vi "Get Section.vi"(11 "Device Info in":refnum<class "Device Info.lvclass">) -> (2 "Section":string, 3 "Device Info out":refnum<class "Device Info.lvclass">)   [LabVIEW 2024, in "EDS.lvlib" / "Device Info.lvclass"]
uses:
  Device Info.lvclass
  Device Info.lvclass/Device Info.ctl
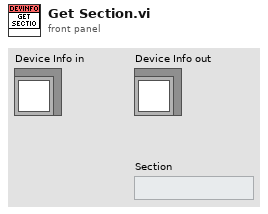
[diagram p1: front panel]
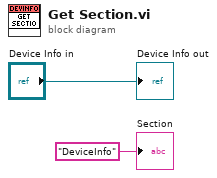
[diagram p0: block diagram]
diagram:
  "Device Info out" <- "Device Info in"
  "Section" <- "DeviceInfo"
